vi "Stop Core.vi"(10 "final error code":i32, 11 "Create Sensor View in":refnum<class "Create Sensor View.lvclass">) -> (3 "Create Sensor View out":refnum<class "Create Sensor View.lvclass">)   [LabVIEW 2013, in "Create Sensor View.lvlib" / "Create Sensor View.lvclass"]
doc: "(<B>Filename</B>: Actor Framework.lvlib:Actor.lvclass:Stop Core.vi)\n\nDefines what the actor does before it stops. Use the <B>final error code</B> input to determine whether the actor shut down in response to an error.\n\nBy default, this method does nothing. A descendant class may override it to define behavior, such as shutting down any processes the actor initiated in its override of the Actor Core method."
uses:
  Create Sensor View.lvclass
  <vilib>/ActorFrameworkMVC/View Actor/View Actor.lvclass
  Create Sensor View.lvclass/Create Sensor View.ctl
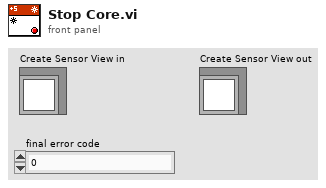
[diagram p1: front panel]
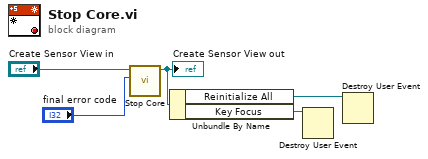
[diagram p0: block diagram]
diagram:
  n1 = call-parent "Stop Core.vi"("final error code"="final error code", "Actor in"="Create Sensor View in") -> ("Actor out"=w3:refnum<class "Create Sensor View.lvclass">)  [unwired: 9 in]
  "Create Sensor View out" <- w3
  n2 = Unbundle By Name(w3) -> ("Reinitialize All"=w2:refnum<user-event>, "Key Focus"=w1:refnum<user-event>)
  n3 = Destroy User Event(user event=w1) -> ()  [unwired: 1 in, 1 out]
  n4 = Destroy User Event(user event=w2) -> ()  [unwired: 1 in, 1 out]
